vi "ConfigFile_ReadEnum.vi"(7 "CFG.SectionName":string, 8 "error in (no error)":errorcluster, 9 "Enum.Strings[]":string[](array[string]), 10 "Enum.Label":string, 11 "ConfigFileRef":T1) -> (0 "error out":errorcluster, 2 "found?":bool, 3 "ConfigFileRef.DUP":T1, 5 "EnumSelection.Out":string)   [LabVIEW 2024]
doc: "Reads a string configuration entry from the configuration file pointed to by <B>configFileRef</B> and converts it to an index as found in <B>enumStrings</B>, which should be the array returned from the Strings[] property of an enumerated data type. The returned index should be fed to the enumerated type, which is used to set its value. An error is returned if the string read from the file is not found in <B>enumStrings</B>.\n_______________________________________________________\n\nPROPRIETARY INFO:\n**********************\nThis software is the property of and contains proprietary information owned by Westinghouse Electric Company and/or its subcontractors and suppliers. It is transmitted to you in confidence and trust, and you agree to treat this software in strict accordance with the terms and conditions of the agreement under which it is provided to you. \n\n© 2011 Westinghouse Electric Company, LLC All rights reserved."
uses:
  <vilib>/Utility/config.llb/Config Data RefNum.ctl
  <vilib>/Utility/config.llb/Read Key (String).vi
  <vilib>/Utility/config.llb/NI_LVConfig.lvlib
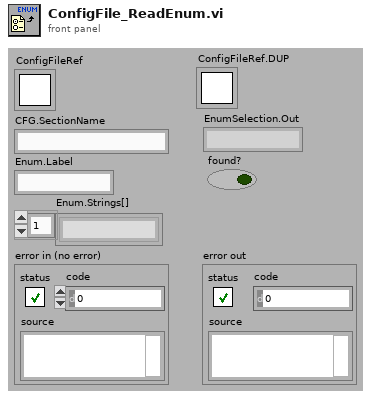
[diagram p1: front panel]
types:
  T1 = typedef "NI_LVConfig.lvlib/Config Data RefNum.ctl" = refnum<k1>
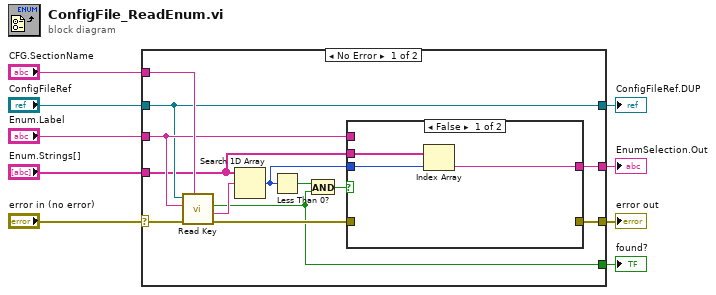
[diagram p0: block diagram]
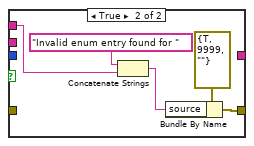
[diagram p2: hidden frame]
diagram:
  n1 = case shown="No Error" "error in (no error)" {
    selector: "error in (no error)" -> [w14 w31]
    tunnel: "ConfigFileRef" -> [w13 _]
    tunnel: "CFG.SectionName" -> [w22 _]
    tunnel: "Enum.Label" -> [w18 _]
    tunnel: [w19 w31] -> w6
    tunnel: [w16 _] -> w5
    tunnel: "Enum.Strings[]" -> [w12 _]
    tunnel: [w13 _] -> w2
    tunnel: [w10 _] -> w1
    frame No Error {
      n2 = call-poly <vilib>:"Read Key.vi"("section"=w22, "error in (no error)"=w14, "key"=w18, "refnum"=w13) -> ("error out"=w20:errorcluster, "value"=w21:string, "found?"=w16:bool)  [unwired: 4 in, 1 out]
      n3 = Search 1D Array(1D array=w12, element=w21) -> (index of element=w11:i32)  [unwired: 1 in]
      n4 = Less Than 0?(x=w11) -> (x < 0?=w17:bool)
      n5 = And(x=w17, y=w16) -> (x .and. y?=w15:bool)
      n6 = case shown="False" w15 {
        tunnel: w20 -> [_ _]
        tunnel: [_ w30] -> w19
        tunnel: w18 -> [_ w28]
        tunnel: w12 -> [w25 _]
        tunnel: w11 -> [w24 _]
        tunnel: [w23 _] -> w10
        frame False {
          n7 = Index Array(array=w25, index=w24) -> (element=w23:string)
        }
        frame True {
          n8 = Concatenate Strings("Invalid enum entry found for " ("source"), w28) -> (w29:string)
          n9 = Bundle By Name(cluster=errorcluster {"status"=TRUE, "code"=9999, "source"=""} ("error out 2"), "source"=w29) -> (w30:errorcluster)
        }
      }
    }
    frame Error {
    }
  }
  "error out" <- w6
  "found?" <- w5
  "ConfigFileRef.DUP" <- w2
  "EnumSelection.Out" <- w1
